vi "ADIS16448_RoboRIO_Teensy_GetSetRefNum.vi"(8 "error in (no error)":errorcluster, 9 "menu":enum16{"set", "get"}(ring), 10 "refnum name":string, 11 "SerialPortRef":T1) -> (0 "error out":errorcluster, 3 "SerialPortRefOut":T1)   [LabVIEW 2016, in "RoboRIO-Teensy-ADIS16448-Interface.lvlib"]
uses:
  RoboRIO-Teensy-ADIS16448-Interface.lvlib
  <vilib>/Rock Robotics/WPI/SerialPort/WPI_SerialPortRef.ctl
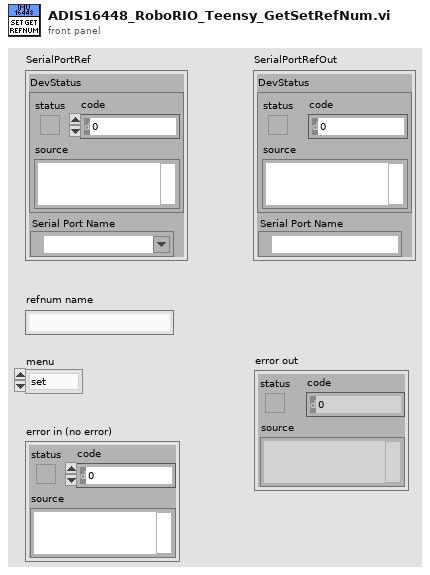
[diagram p1: front panel]
types:
  T1 = typedef "WPI_SerialPortRef.ctl" = cluster{"DevStatus":errorcluster, "Serial Port Name":refnum<visa-resource-name>}
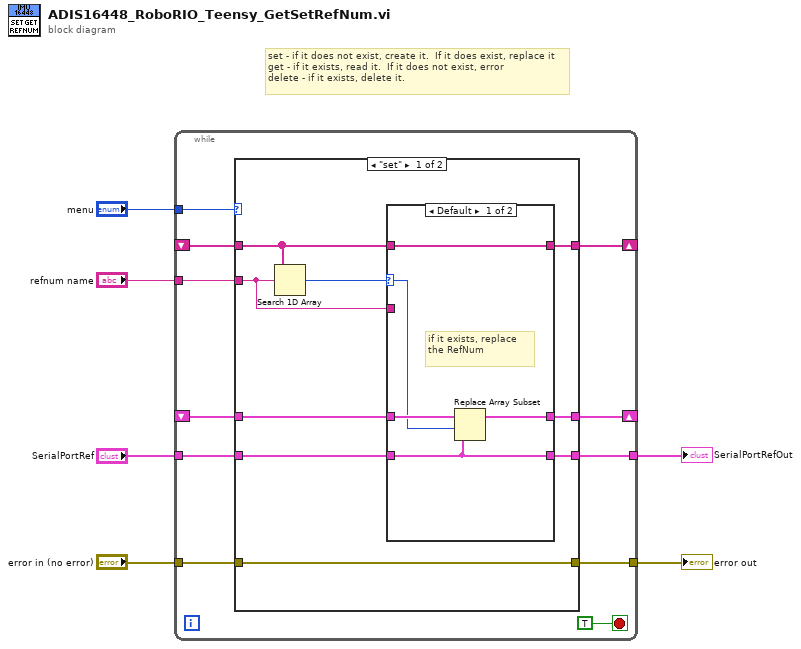
[diagram p0: block diagram]
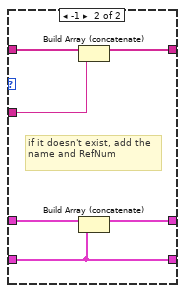
[diagram p2: hidden frame]
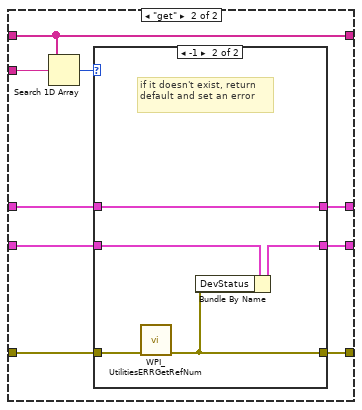
[diagram p3: hidden frame]
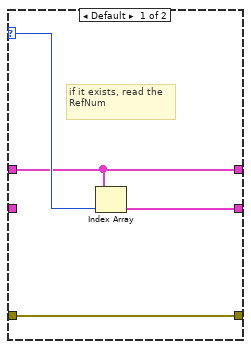
[diagram p4: hidden frame]
diagram:
  # "set - if it does not exist, create it.  If it does exist, replace it\nget - if it exists, read it.  If it does not exist, error\ndelete - if it exists, delete it."
  n1 = while {
    tunnel: "SerialPortRef" -> [w17]
    tunnel: "refnum name" -> [w10]
    tunnel: "error in (no error)" -> [w9]
    shift-right: [w16] -> _
    shift-left: _ -> [w15]
    tunnel: [w14] -> w1
    tunnel: "menu" -> [w13]
    shift-right: [w12] -> _
    shift-left: _ -> [w11]
    tunnel: [w8] -> w4
    stop <- TRUE stop-if-true
    n2 = case shown="\"set\"" w13 {
      tunnel: w17 -> [w21 w43]
      tunnel: [w20 w42] -> w16
      tunnel: w15 -> [w22 w44]
      tunnel: [w19 w41] -> w14
      tunnel: [w26 w40] -> w12
      tunnel: w11 -> [w25 w40]
      tunnel: w10 -> [w23 w45]
      tunnel: [w18 w38] -> w8
      tunnel: w9 -> [w18 w39]
      frame "set" {
        n3 = Search 1D Array(1D array=w25, element=w23) -> (index of element=w24:i32)  [unwired: 1 out]
        n4 = case shown="Default" w24 {
          selector: w24 -> [w29 _]
          tunnel: [w31 w37] -> w26
          tunnel: w25 -> [w31 w36]
          tunnel: w23 -> [_ w35]
          tunnel: w22 -> [w30 w34]
          tunnel: w21 -> [w27 w32]
          tunnel: [w28 w33] -> w20
          tunnel: [w27 w32] -> w19
          frame Default {
            # "if it exists, replace the RefNum"
            n5 = Replace Array Subset(array=w30, new element=w27, index=w29) -> (w28:T1[])
          }
          frame -1 {
            # "if it doesn't exist, add the name and RefNum"
            n6 = Build Array (concatenate)(w36, w35) -> (w37:string[])
            n7 = Build Array (concatenate)(w34, w32) -> (w33:T1[])
          }
        }
      }
      frame "get" {
        n8 = Search 1D Array(1D array=w40, element=w45) -> (index of element=w46:i32)  [unwired: 1 out]
        n9 = case shown="-1" w46 {
          selector: w46 -> [w50 _]
          tunnel: w44 -> [w48 w55]
          tunnel: w43 -> [_ w53]
          tunnel: [w48 w55] -> w42
          tunnel: [w49 w52] -> w41
          tunnel: w39 -> [w47 w54]
          tunnel: [w47 w51] -> w38
          frame Default {
            # "if it exists, read the RefNum"
            n10 = Index Array(array=w48, index=w50) -> (element=w49:T1)
          }
          frame -1 {
            # "if it doesn't exist, return default and set an error"
            n11 = call <vilib>:"WPI_UtilitiesERRGetRefNum.vi"("error in (no error)"=w54) -> ("ERRGetRefNum"=w51:errorcluster)  [unwired: 10 out]
            n12 = Bundle By Name(cluster=w53, "DevStatus"=w51) -> (w52:T1)
          }
        }
      }
    }
  }
  "error out" <- w4
  "SerialPortRefOut" <- w1
